vi "COM CUST -Append Rest Param Vals.vi"(0 "DBParmKey|Value":string[][](array[string]), 2 "LclParamVal":string[][](array[string])) -> (14 "AllParamvalue":string[][](array[string]))   [LabVIEW 2019]
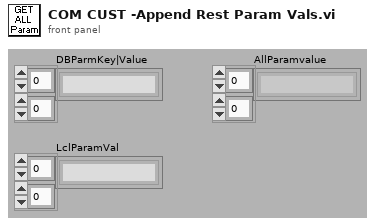
[diagram p1: front panel]
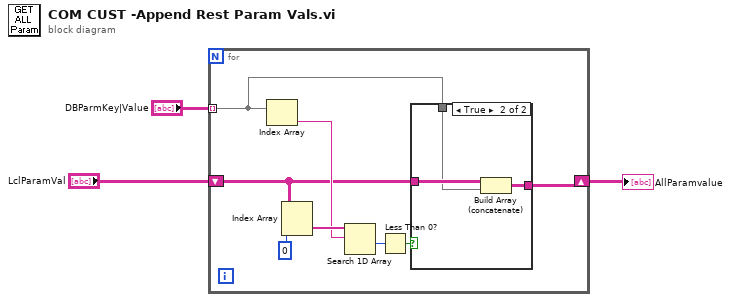
[diagram p0: block diagram]
diagram:
  n1 = for {
    tunnel: "DBParmKey|Value" -> [w6] mode=indexing
    shift-right: [w4] -> w1
    shift-left: "LclParamVal" -> [w5]
    n2 = Index Array(array=w6) -> (element=w9:string)  [unwired: 1 in]
    n3 = Index Array(array=w5, index (col)=0 ("disabled index (col)")) -> (element=w10:string[])  [unwired: 1 in]
    n4 = Search 1D Array(1D array=w10, element=w9) -> (index of element=w8:i32)  [unwired: 1 out]
    n5 = Less Than 0?(x=w8) -> (x < 0?=w7:bool)
    n6 = case shown="True" w7 {
      tunnel: w6 -> [_ w13]
      tunnel: w5 -> [w12 w15]
      tunnel: [w12 w14] -> w4
      frame False {
      }
      frame True {
        n7 = Build Array (concatenate)(w15, w13) -> (w14:string[][])
      }
    }
  }
  "AllParamvalue" <- w1
